vi "Display EtherCAT Provider Error.vi"(8 "error in":errorcluster) -> (0 "error out":errorcluster)   [LabVIEW 2019, in "SEECD System Explorer.lvlib"]
uses:
  SEECD System Explorer.lvlib
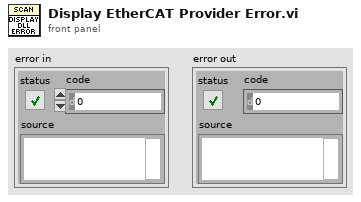
[diagram p1: front panel]
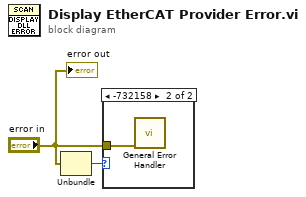
[diagram p0: block diagram]
diagram:
  n1 = Unbundle("error in") -> ("code"=w2:i32)  [unwired: 2 out]
  n2 = case shown="-732158" w2 {
    tunnel: "error in" -> [_ w3]
    frame 0, Default {
    }
    frame -732158 {
      n3 = call <vilib>:"General Error Handler.vi"("error in (no error)"=w3) -> ()  [unwired: 10 in, 5 out]
    }
  }
  "error out" <- "error in"
